vi "Function.vi"(8 "error in (no error)":errorcluster, 10 "Numeric":T1, 11 "Two Terminal in":refnum<class "Not Equal 0_U64.lvclass">) -> (0 "error out":errorcluster, 2 "Result":bool, 3 "Two Terminal out":refnum<class "Not Equal 0_U64.lvclass">)   [LabVIEW 2021, in "Not Equal 0_U64.lvclass"]
uses:
  Not Equal 0_U64.lvclass
  Support/Compare/One Term/U64/Support/Data Type.ctl
  Support/Compare/One Term/U64/AbsComp_One Term_U64.lvclass
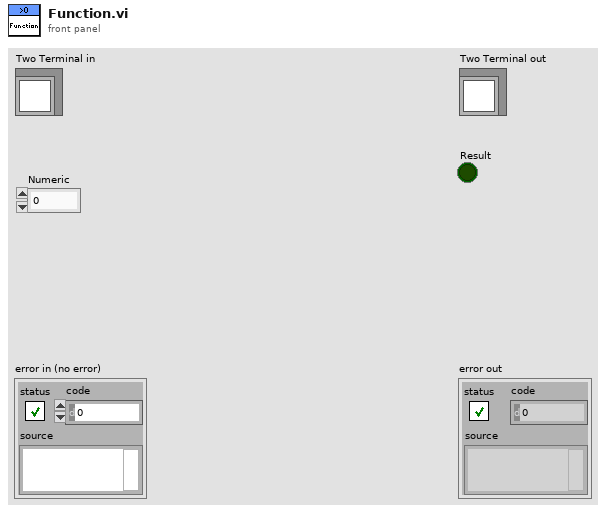
[diagram p1: front panel]
types:
  T1 = typedef "AbsComp_One Term_U64.lvclass/Data Type.ctl" = u64
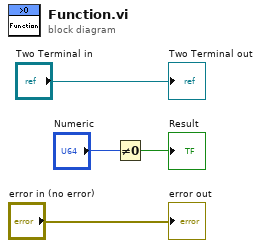
[diagram p0: block diagram]
diagram:
  n1 = Not Equal To 0?(x="Numeric") -> (x != 0?=→"Result":bool)
  "error out" <- "error in (no error)"
  "Two Terminal out" <- "Two Terminal in"
